vi "Lockin_SR830_readXY.vi"(2 "Variable":string="1,2", 3 "VISA Resource Name":refnum<visa-resource-name>="GPIB0::8::INSTR") -> (0 "Output Y":dbl, 1 "Output X":dbl)   [LabVIEW 2011]
panel:
  # "Variable : \n1=X\n2=Y\n3=R\n4=theta\nis added to the command \nOUTP?"
  # "always put 1 pairs of variable"
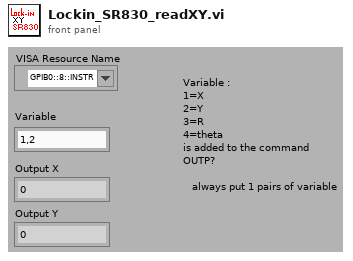
[diagram p1: front panel]
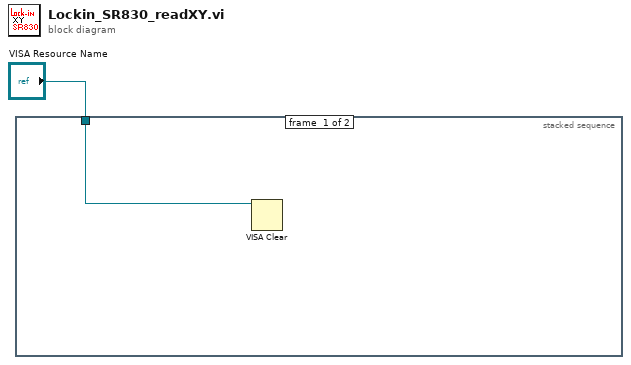
[diagram p0: block diagram]
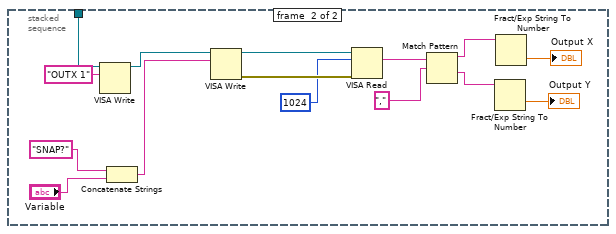
[diagram p2: hidden frame]
diagram:
  n1 = stacked-sequence {
    tunnel: "VISA Resource Name" -> [w2 w3]
    frame #0 {
      n2 = VISA Clear(VISA resource name=w2) -> ()  [unwired: 1 in, 2 out]
    }
    frame #1 {
      n3 = VISA Write(VISA resource name=w3, write buffer="OUTX 1") -> (VISA resource name out=w5:refnum<visa-resource-name>)  [unwired: 1 in, 2 out]
      n4 = Concatenate Strings("SNAP?" ("Command"), "Variable") -> (w13:string)
      n5 = VISA Write(VISA resource name=w5, write buffer=w13) -> (VISA resource name out=w17:refnum<visa-resource-name>, error out=w16:errorcluster)  [unwired: 1 in, 1 out]
      n6 = VISA Read(VISA resource name=w17, byte count=1024, error in (no error)=w16) -> (read buffer=w11:string)  [unwired: 3 out]
      n7 = Match Pattern(string=w11, regular expression=",") -> (before substring=w9:string, after substring=w7:string)  [unwired: 1 in, 2 out]
      n8 = Fract/Exp String To Number(string=w7) -> (number=→"Output Y":dbl)  [unwired: 3 in, 1 out]
      n9 = Fract/Exp String To Number(string=w9) -> (number=→"Output X":dbl)  [unwired: 3 in, 1 out]
    }
  }
